vi "Read.vi"(7 "Read Type":T1, 8 "error in (no error)":errorcluster, 11 "NetworkStreamReader in":refnum<class "NetworkStreamReader.lvclass">) -> (0 "error out":errorcluster, 1 "New element?":bool, 2 "element":variant, 3 "NetworkStreamReader out":refnum<class "NetworkStreamReader.lvclass">, 4 "Time Stamp":timestamp)   [LabVIEW 2013, in "NetworkStreamReader.lvclass"]
doc: "Returns the requested value (either the next element available in the buffer or the most recent element). If there are no elements available in the queue, this VI will return the last valid value it returned.\n\nJared Kirschner, 2012."
uses:
  NetworkStreamReader.lvclass
  readType.ctl
  NetworkStreamReader.lvclass/NetworkStreamReader.ctl
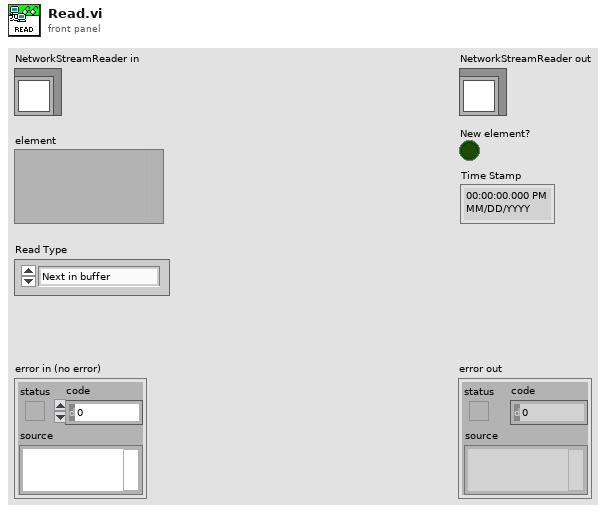
[diagram p1: front panel]
types:
  T1 = typedef "NetworkStreamReader.lvclass/readType.ctl" = enum16{"Next in buffer", "Most current"}
  T2 = typedef "TimeStampedMessageQueue.ctl" = refnum<queue>
  T3 = typedef "TimeStampedMessage.ctl" = cluster{"Data":variant, "Time Stamp":timestamp}
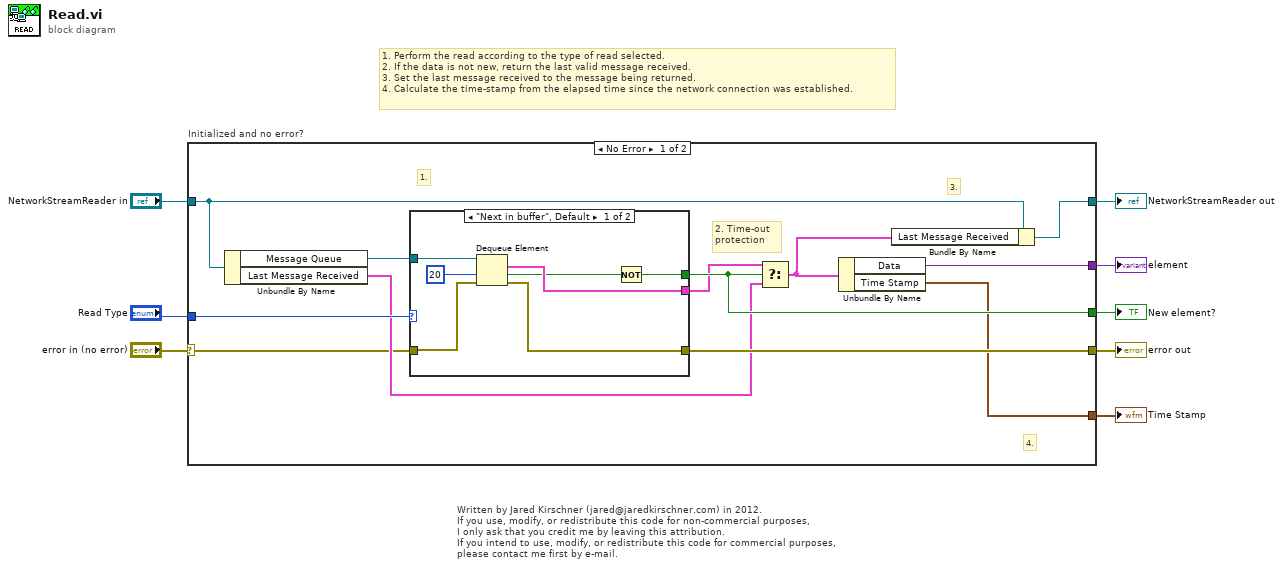
[diagram p0: block diagram]
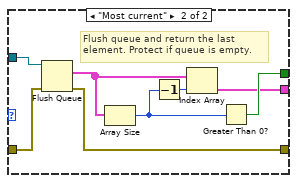
[diagram p2: hidden frame]
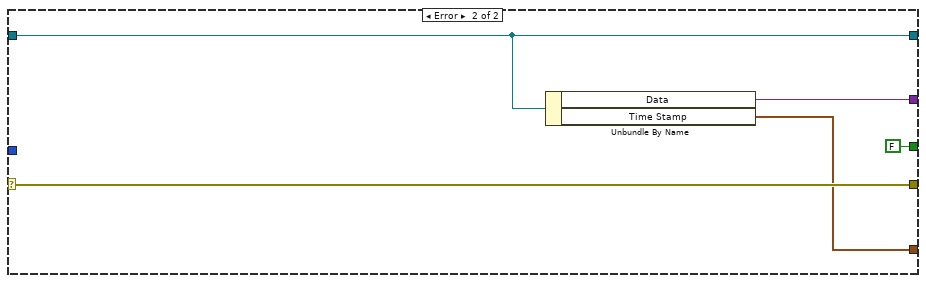
[diagram p3: hidden frame]
diagram:
  # "1. Perform the read according to the type of read selected.\n2. If the data is not new, return the last valid message received.\n3. Set the last message received to the message being returned.\n4. Calculate the time-stamp from the elapsed time since the network connection was established."
  # "Written by Jared Kirschner (jared@jaredkirschner.com) in 2012.\nIf you use, modify, or redistribute this code for non-commercial purposes,\nI only ask that you credit me by leaving this attribution.\nIf you intend to use, modify, or redistribute this code for commercial purposes,\nplease contact me first by e-mail."
  n1 = case "Initialized and no error?" shown="No Error" "error in (no error)" {
    selector: "error in (no error)" -> [w10 w37]
    tunnel: [w19 w37] -> w8
    tunnel: [w16 w40] -> w7
    tunnel: "NetworkStreamReader in" -> [w17 w40]
    tunnel: [w13 w39] -> w6
    tunnel: "Read Type" -> [w18 _]
    tunnel: [w15 FALSE] -> w4
    tunnel: [w9 w36] -> w3
    frame No Error {
      # "4."
      # "3."
      # "1."
      # "2. Time-out \nprotection"
      n2 = Unbundle By Name(w17) -> ("Message Queue"=w20:T2, "Last Message Received"=w11:T3)
      n3 = case shown="\"Next in buffer\", Default" w18 {
        tunnel: w20 -> [w27 w35]
        tunnel: [w24 w32] -> w19
        tunnel: w10 -> [w25 w34]
        tunnel: [w22 w33] -> w15
        tunnel: [w23 w28] -> w12
        frame "Next in buffer", Default {
          n4 = Dequeue Element(queue=w27, timeout in ms (-1)=20, error in (no error)=w25) -> (element=w23:T3, timed out?=w21:bool, error out=w24:errorcluster)  [unwired: 1 out]
          n5 = Not(x=w21) -> (.not. x?=w22:bool)
        }
        frame "Most current" {
          # "Flush queue and return the last\nelement. Protect if queue is empty."
          n6 = Flush Queue(queue=w35, error in (no error)=w34) -> (remaining elements=w30:T3[], error out=w32:errorcluster)  [unwired: 1 out]
          n7 = Array Size(array=w30) -> (size(s)=w31:i32)
          n8 = Decrement(x=w31) -> (x-1=w29:i32)
          n9 = Index Array(array=w30, index=w29) -> (element=w28:T3)
          n10 = Greater Than 0?(x=w31) -> (x > 0?=w33:bool)
        }
      }
      n11 = Select(t=w12, s=w15, f=w11) -> (s? t:f=w14:T3)
      n12 = Unbundle By Name(w14) -> ("Data"=w13:variant, "Time Stamp"=w9:timestamp)
      n13 = Bundle By Name(cluster=w17, "Last Message Received"=w14) -> (w16:refnum<class "NetworkStreamReader.lvclass">)
    }
    frame Error {
      n14 = Unbundle By Name(w40) -> ("Data"=w39:variant, "Time Stamp"=w36:timestamp)
    }
  }
  "error out" <- w8
  "NetworkStreamReader out" <- w7
  "element" <- w6
  "New element?" <- w4
  "Time Stamp" <- w3
